vi "transfer product_manual.vi"() -> ()   [LabVIEW 2023]
uses:
  <vilib>/DAQmx/read.llb/DAQmx Read (Digital 1D Bool 1Chan 1Samp).vi
  <vilib>/DAQmx/create/channels.llb/DAQmx Create Channel (DI-Digital Input).vi
  <vilib>/DAQmx/miscellaneous.llb/DAQmx Fill In Error Info.vi
panel:
  out "sensor":bool[](array[boolean])
  in  "stop":bool
  in  "index":i8
  in  "channel":i8
  out "channel":string
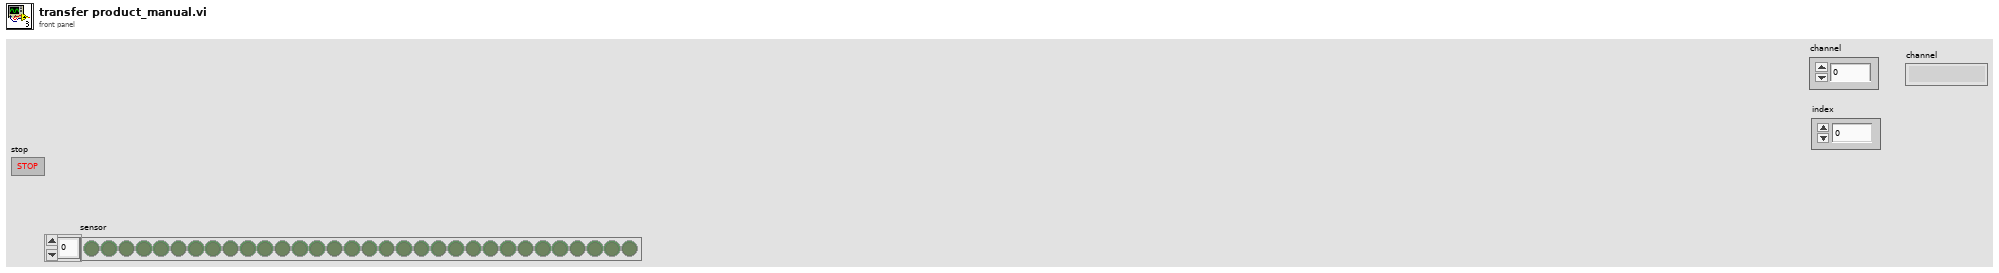
[diagram p1: front panel]
types:
  T1 = enum16{"plate1", "plate2", "plate3", "rinse", "seat"}
  T2 = enum16{"Initialize", "Absolute Position", "Relative Pickup", "Relative Dispense", "Swich valve", "Bypass"}
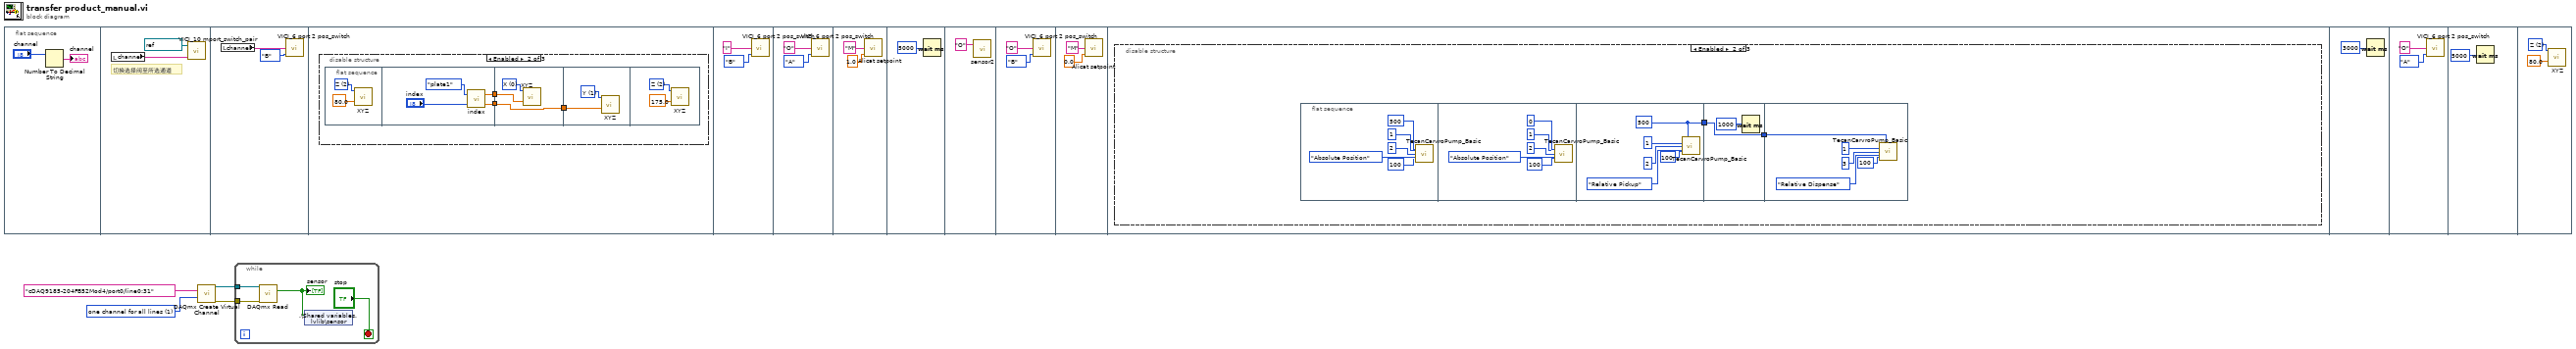
[diagram p0: block diagram]
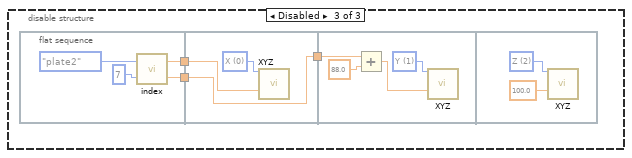
[diagram p3: hidden frame]
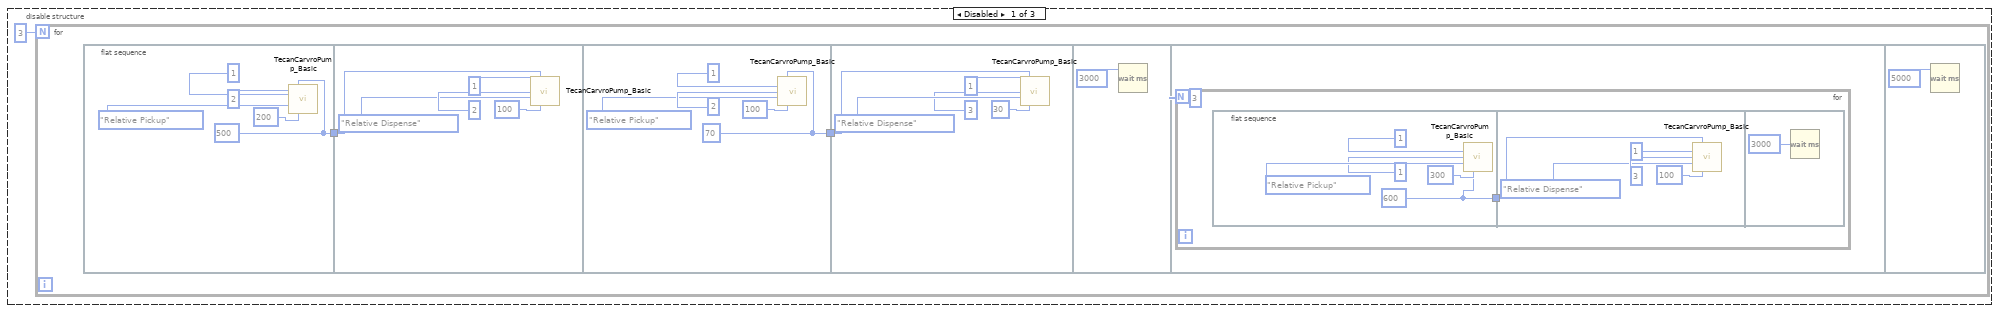
[diagram p4: hidden frame]
diagram:
  w4 = 1 items=["one channel for each line", "one channel for all lines"] ("line grouping")
  n1 = flat-sequence {
    frame #0 {
      n2 = Number To Decimal String(number="channel") -> (decimal integer string=→"channel":string)  [unwired: 1 in]
    }
    frame #1 {
      # "切换选择阀至所选通道"
      n3 = local read "channel"() -> (w8:string)
      n4 = call "VICI_10 mport_switch_pair.vi"("Go to position"=w8, "Valve COM"=refnum<visa-resource-name> "COM8") -> ()  [unwired: 2 in, 1 out]
    }
    frame #2 {
      n5 = local read "channel"() -> (w10:string)
      n6 = call "VICI_6 port 2 pos_switch.vi"("Switch to position (A/B)"=enum16{"A", "B"}."B", "Valve ID"=w10) -> ()  [unwired: 2 in, 1 out]
    }
    frame #3 {
      n7 = disable-structure shown="Enabled" {
        frame Disabled {
        }
        frame Enabled {
          n8 = flat-sequence {
            tunnel: [w18] -> w13
            tunnel: [w17] -> w12
            tunnel: w13 -> [w20]
            tunnel: w12 -> [w22]
            tunnel: [w22] -> w11
            tunnel: w11 -> [w23]
            frame #0 {
              w14 = u16 2 items=["X", "Y", "Z"] ("AXIS")
              n9 = call "XYZ.vi"("AXIS"=w14, "Set location (mm)"=80.0) -> ()  [unwired: 9 in, 5 out]
            }
            frame #1 {
              n10 = call "index.vi"("index"="index", "where"=T1."plate1") -> ("Y"=w17:dbl, "X"=w18:dbl)
            }
            frame #2 {
              w21 = u16 0 items=["X", "Y", "Z"] ("AXIS")
              n11 = call "XYZ.vi"("AXIS"=w21, "Set location (mm)"=w20) -> ()  [unwired: 9 in, 5 out]
            }
            frame #3 {
              w24 = u16 1 items=["X", "Y", "Z"] ("AXIS")
              n12 = call "XYZ.vi"("AXIS"=w24, "Set location (mm)"=w23) -> ()  [unwired: 9 in, 5 out]
            }
            frame #4 {
              w26 = u16 2 items=["X", "Y", "Z"] ("AXIS")
              n13 = call "XYZ.vi"("AXIS"=w26, "Set location (mm)"=175.0) -> ()  [unwired: 9 in, 5 out]
            }
          }
        }
        frame Disabled {
          n14 = flat-sequence {
            tunnel: [w31] -> w29
            tunnel: [w30] -> w27
            tunnel: w29 -> [w35]
            tunnel: [w34] -> w28
            tunnel: w27 -> [w34]
            tunnel: w28 -> [w37]
            frame #0 {
              n15 = call "index.vi"("index"=i8 7, "where"=T1."plate2") -> ("Y"=w30:dbl, "X"=w31:dbl)
            }
            frame #1 {
              w36 = u16 0 items=["X", "Y", "Z"] ("AXIS")
              n16 = call "XYZ.vi"("AXIS"=w36, "Set location (mm)"=w35) -> ()  [unwired: 9 in, 5 out]
            }
            frame #2 {
              w39 = u16 1 items=["X", "Y", "Z"] ("AXIS")
              n17 = Add(x=w37, y=88.0) -> (x+y=w40:dbl)
              n18 = call "XYZ.vi"("AXIS"=w39, "Set location (mm)"=w40) -> ()  [unwired: 9 in, 5 out]
            }
            frame #3 {
              w42 = u16 2 items=["X", "Y", "Z"] ("AXIS")
              n19 = call "XYZ.vi"("AXIS"=w42, "Set location (mm)"=100.0) -> ()  [unwired: 9 in, 5 out]
            }
          }
        }
      }
    }
    frame #4 {
      n20 = call "VICI_6 port 2 pos_switch.vi"("Switch to position (A/B)"=enum16{"A", "B"}."B", "Valve ID"="I") -> ()  [unwired: 2 in, 1 out]
    }
    frame #5 {
      n21 = call "VICI_6 port 2 pos_switch.vi"("Switch to position (A/B)"=enum16{"A", "B"}."A", "Valve ID"="O") -> ()  [unwired: 2 in, 1 out]
    }
    frame #6 {
      n22 = call "Alicat setpoint.vi"("Setpoint"=1.0, "Unit ID"="M") -> ()  [unwired: 3 in]
    }
    frame #7 {
      n23 = Wait (ms)(milliseconds to wait=u32 5000) -> ()  [unwired: 1 out]
    }
    frame #8 {
      n24 = call "sensor2.vi"("Sensor"="O") -> ()  [unwired: 1 in, 2 out]
    }
    frame #9 {
      n25 = call "VICI_6 port 2 pos_switch.vi"("Switch to position (A/B)"=enum16{"A", "B"}."B", "Valve ID"="O") -> ()  [unwired: 2 in, 1 out]
    }
    frame #10 {
      n26 = call "Alicat setpoint.vi"("Setpoint"=0.0, "Unit ID"="M") -> ()  [unwired: 3 in]
    }
    frame #11 {
      n27 = disable-structure shown="Enabled" {
        frame Disabled {
          n28 = for {
            N: 3 -> [_]
            n29 = flat-sequence {
              tunnel: [w58] -> w57
              tunnel: w57 -> [w63]
              tunnel: [w68] -> w56
              tunnel: w56 -> [w73]
              frame #0 {
                w58 = u16 500 ("Volume (μL)")
                n30 = call "TecanCarvroPump_Basic.vi"("Volume (μL)"=w58, "TecanPump address"=u8 1, "Valve"=u8 2, "Mode"=T2."Relative Pickup", "Speed (μL/s)"=u16 200) -> ()  [unwired: 10 in, 1 out]
              }
              frame #1 {
                n31 = call "TecanCarvroPump_Basic.vi"("Volume (μL)"=w63, "TecanPump address"=u8 1, "Valve"=u8 2, "Mode"=T2."Relative Dispense", "Speed (μL/s)"=u16 100) -> ()  [unwired: 10 in, 1 out]
              }
              frame #2 {
                w68 = u16 70 ("Volume (μL)")
                n32 = call "TecanCarvroPump_Basic.vi"("Volume (μL)"=w68, "TecanPump address"=u8 1, "Valve"=u8 2, "Mode"=T2."Relative Pickup", "Speed (μL/s)"=u16 100) -> ()  [unwired: 10 in, 1 out]
              }
              frame #3 {
                n33 = call "TecanCarvroPump_Basic.vi"("Volume (μL)"=w73, "TecanPump address"=u8 1, "Valve"=u8 3, "Mode"=T2."Relative Dispense", "Speed (μL/s)"=u16 30) -> ()  [unwired: 10 in, 1 out]
              }
              frame #4 {
                n34 = Wait (ms)(milliseconds to wait=u32 3000) -> ()  [unwired: 1 out]
              }
              frame #5 {
                n35 = for {
                  N: 3 -> [_]
                  n36 = flat-sequence {
                    tunnel: [w81] -> w80
                    tunnel: w80 -> [w86]
                    frame #0 {
                      w81 = u16 600 ("Volume (μL)")
                      n37 = call "TecanCarvroPump_Basic.vi"("Volume (μL)"=w81, "TecanPump address"=u8 1, "Valve"=u8 1, "Mode"=T2."Relative Pickup", "Speed (μL/s)"=u16 300) -> ()  [unwired: 10 in, 1 out]
                    }
                    frame #1 {
                      n38 = call "TecanCarvroPump_Basic.vi"("Volume (μL)"=w86, "TecanPump address"=u8 1, "Valve"=u8 3, "Mode"=T2."Relative Dispense", "Speed (μL/s)"=u16 100) -> ()  [unwired: 10 in, 1 out]
                    }
                    frame #2 {
                      n39 = Wait (ms)(milliseconds to wait=u32 3000) -> ()  [unwired: 1 out]
                    }
                  }
                }
              }
              frame #6 {
                n40 = Wait (ms)(milliseconds to wait=u32 5000) -> ()  [unwired: 1 out]
              }
            }
          }
        }
        frame Enabled {
          n41 = flat-sequence {
            tunnel: [w105] -> w94
            tunnel: w94 -> [w111]
            tunnel: [w111] -> w93
            tunnel: w93 -> [w112]
            frame #0 {
              n42 = call "TecanCarvroPump_Basic.vi"("Volume (μL)"=u16 500, "TecanPump address"=u8 1, "Valve"=u8 2, "Mode"=T2."Absolute Position", "Speed (μL/s)"=u16 100) -> ()  [unwired: 10 in, 1 out]
            }
            frame #1 {
              n43 = call "TecanCarvroPump_Basic.vi"("Volume (μL)"=u16 0, "TecanPump address"=u8 1, "Valve"=u8 2, "Mode"=T2."Absolute Position", "Speed (μL/s)"=u16 100) -> ()  [unwired: 10 in, 1 out]
            }
            frame #2 {
              w105 = u16 500 ("Volume (μL)")
              n44 = call "TecanCarvroPump_Basic.vi"("Volume (μL)"=w105, "TecanPump address"=u8 1, "Valve"=u8 2, "Mode"=T2."Relative Pickup", "Speed (μL/s)"=u16 100) -> ()  [unwired: 10 in, 1 out]
            }
            frame #3 {
              n45 = Wait (ms)(milliseconds to wait=u32 1000) -> ()  [unwired: 1 out]
            }
            frame #4 {
              n46 = call "TecanCarvroPump_Basic.vi"("Volume (μL)"=w112, "TecanPump address"=u8 1, "Valve"=u8 3, "Mode"=T2."Relative Dispense", "Speed (μL/s)"=u16 100) -> ()  [unwired: 10 in, 1 out]
            }
          }
        }
        frame Disabled {
        }
      }
    }
    frame #12 {
      n47 = Wait (ms)(milliseconds to wait=u32 3000) -> ()  [unwired: 1 out]
    }
    frame #13 {
      n48 = call "VICI_6 port 2 pos_switch.vi"("Switch to position (A/B)"=enum16{"A", "B"}."A", "Valve ID"="O") -> ()  [unwired: 2 in, 1 out]
    }
    frame #14 {
      n49 = Wait (ms)(milliseconds to wait=u32 5000) -> ()  [unwired: 1 out]
    }
    frame #15 {
      w122 = u16 2 items=["X", "Y", "Z"] ("AXIS")
      n50 = call "XYZ.vi"("AXIS"=w122, "Set location (mm)"=80.0) -> ()  [unwired: 9 in, 5 out]
    }
  }
  n51 = call-poly <vilib>:"DAQmx Create Virtual Channel.vi"("lines"=tag "cDAQ9185-204FB52Mod4/port0/line0:31", "line grouping"=w4) -> ("task out"=w3:refnum<k21>, "error out"=w2:errorcluster)  [unwired: 12 in]
  n52 = while {
    tunnel: w3 -> [w126]
    tunnel: w2 -> [w125]
    stop <- "stop" stop-if-true
    n53 = call-poly <vilib>:"DAQmx Read.vi"("task/channels in"=w126, "error in"=w125) -> ("data"=w124:bool[])  [unwired: 11 in, 2 out]
    "sensor" <- w124
    n54 = shared-variable ".\\Shared variables.lvlib\\sensor"(w124) -> ()  [unwired: 1 in, 1 out]
  }
